vi "Template Dut TxRx Abort.vi"(0 "Dut Handle in":T1, 7 "Tx?":bool, 11 "error in (no error)":errorcluster) -> (4 "Dut Handle out":T1, 15 "error out":errorcluster)   [LabVIEW 2014, in "niDTS Template.lvlib"]
uses:
  niDTS Template.lvlib
  Framework/Dut/Includes/niDTS Dut INC Handle.ctl
  Framework/Dut/Objects/BASE_class/niDTS Dut.lvclass
  Includes/Template Dut INC Handle.ctl
  Objects/BASE_class/Template Dut.lvclass
  Framework/niDTS Framework.lvlib
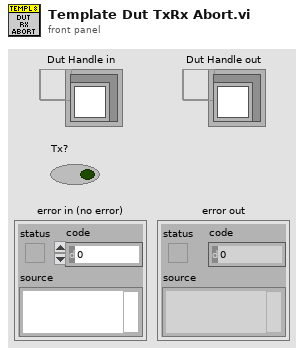
[diagram p1: front panel]
types:
  T1 = typedef "niDTS Framework.lvlib/niDTS Dut INC Handle.ctl" = refnum<data-value>
  T2 = typedef "niDTS Template.lvlib/Template Dut INC Handle.ctl" = refnum<data-value>
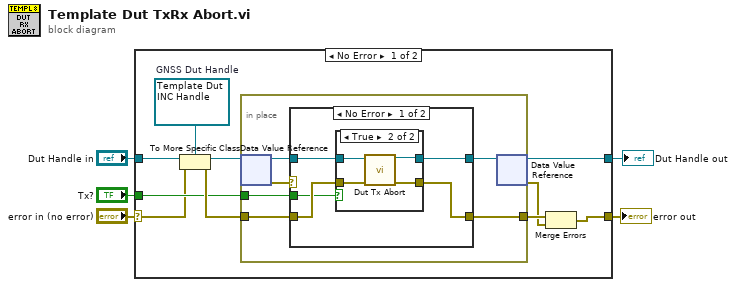
[diagram p0: block diagram]
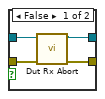
[diagram p2: hidden frame]
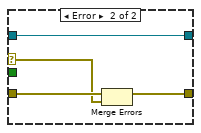
[diagram p3: hidden frame]
diagram:
  n1 = case shown="No Error" "error in (no error)" {
    selector: "error in (no error)" -> [w6 w39]
    tunnel: "Dut Handle in" -> [w15 w40]
    tunnel: [w14 w40] -> w4
    tunnel: [w9 w39] -> w3
    tunnel: "Tx?" -> [w7 _]
    frame No Error {
      w11 = T2 refnum  # GNSS Dut Handle
      n2 = To More Specific Class(target class=w11, reference=w15, error in=w6) -> (specific class reference=w13:T2, error out=w12:errorcluster)
      n3 = in-place {
        in-place-border: w12 -> [w18]
        in-place-border: [w17] -> w10
        in-place-border: w7 -> [w16]
        n4 = in-place-dvr #1(w13) -> (w20:refnum<class "Template Dut.lvclass">, w21:errorcluster)
        n5 = case shown="No Error" w21 {
          selector: w21 -> [_ w36]
          tunnel: w20 -> [w26 w38]
          tunnel: [w25 w38] -> w19
          tunnel: w18 -> [w24 w37]
          tunnel: [w23 w35] -> w17
          tunnel: w16 -> [w22 _]
          frame No Error {
            n6 = case shown="True" w22 {
              tunnel: w26 -> [w30 w33]
              tunnel: [w29 w32] -> w25
              tunnel: w24 -> [w28 w34]
              tunnel: [w27 w31] -> w23
              frame False {
                n7 = call-dynamic "Dut Rx Abort.vi"("niDTS DUT in"=w30, "error in (no error)"=w28) -> ("niDTS DUT out"=w29:refnum<class "Template Dut.lvclass">, "error out"=w27:errorcluster)  [unwired: 12 in]
              }
              frame True {
                n8 = call-dynamic "Dut Tx Abort.vi"("niDTS DUT in"=w33, "error in (no error)"=w34) -> ("niDTS DUT out"=w32:refnum<class "Template Dut.lvclass">, "error out"=w31:errorcluster)  [unwired: 12 in]
              }
            }
          }
          frame Error {
            n9 = Merge Errors(w37, w36) -> (w35:errorcluster)
          }
        }
        n10 = in-place-dvr #1(w19) -> (w14:T2, w8:errorcluster)
      }
      n11 = Merge Errors(w10, w8) -> (w9:errorcluster)
    }
    frame Error {
    }
  }
  "Dut Handle out" <- w4
  "error out" <- w3
